vi "I(V) at various fields_MFLI_PK_v4.0_measure X.vi"() -> ()   [LabVIEW 2016]
uses:
  <instrlib>/Zurich Instruments LabOne/Public/Data/ziTypeDemodSampleSingle.ctl
  <instrlib>/Zurich Instruments LabOne/Public/Configure/ziSetValueDouble.vi
  <instrlib>/Zurich Instruments LabOne/Public/Configure/ziGetValueDemodSampleEx.vi
  <instrlib>/Zurich Instruments LabOne/Zurich Instruments LabOne.lvlib
panel:
  out "Time (s)":dbl format="%#_13g"
  in  "Field ramp rate (T/min)":string="0.05"
  in  "Magnetic field stabilization time (s)":dbl=200.0 format="%#_13g"
  in  "Step 2":dbl[](array[numeric])=[0.25] min=-3000.0 max=3000.0 format="%.1e"
  in  "To 2":dbl[](array[numeric])=[6.0] min=-3000.0 max=3000.0 format="%.1e"
  in  "From 2":dbl[](array[numeric])=[8.5] min=-3000.0 max=3000.0 format="%.1e"
  out "Magnetic Field (T)":dbl format="%#_13g"
  in  "Magnet IP Address":string="169.254.46.132"
  out "Demod Sample Out 2":T1={"Timestamps (ticks)"=34359738372, "X (Vrms)"=8.366245757779461e-285, "Y (Vrms)"=1.0096057436928657e-284, "Osc Phase (deg)"=1.69759663376e-313, "Freq (Hz)"=2.607691286315397e-191, "DIO"=4, "AuxIn0 (V)"=0.0, "AuxIn1 (V)"=1.6954746369817e-311, "Trigger"=16}
  out "Demod Sample Out":T1={"Timestamps (ticks)"=34359738372, "X (Vrms)"=8.366245757779461e-285, "Y (Vrms)"=1.0096057436928657e-284, "Osc Phase (deg)"=1.69759663376e-313, "Freq (Hz)"=2.607691286315397e-191, "DIO"=4, "AuxIn0 (V)"=0.0, "AuxIn1 (V)"=1.6954746369817e-311, "Trigger"=16}
  in  "MFLI Current source/Voltage reader":string="DEV4382"
  out "Imeas (A)":dbl=2.528615115e-315
  out "Vmeas (V)":dbl=nan
  in  "Folder":path=path "D:/Pranava/Data/NbO/27-05-2020"
  in  "MFLI stabilization time (s) [> TC]":u32=1
  out "I vs V":cluster{dbl, "Field Reading":dbl}[](graph)=[{nan, "Field Reading"=3.54694038e-315}, {nan, "Field Reading"=2.528615115e-315}]
  out "data":dbl[](array[numeric])=[nan, 2.528615115e-315, 0.0001]
  in  "Step":dbl[](array[numeric])=[0.001, 0.001, 0.001] min=-3000.0 max=3000.0 format="%.1e"
  in  "To":dbl[](array[numeric])=[0.5, -0.5, 0.0] min=-3000.0 max=3000.0 format="%.1e"
  in  "From":dbl[](array[numeric])=[0.0, 0.5, -0.5] min=-3000.0 max=3000.0 format="%.1e"
  in  "file name":string="001_IV_(Nb)STO_7mK_MFLI_MF-MD"
  out "File path":path=path "D:/Pranava/Data/001_IV_(Nb)STO_7mK_MFLI_MF-MD.dat"
  # ".dat"
  # "[Must be less than 0.05]"
  # "Set MFLI Voltage output (V)"
  # "Configure Magnetic field sweep (T)"
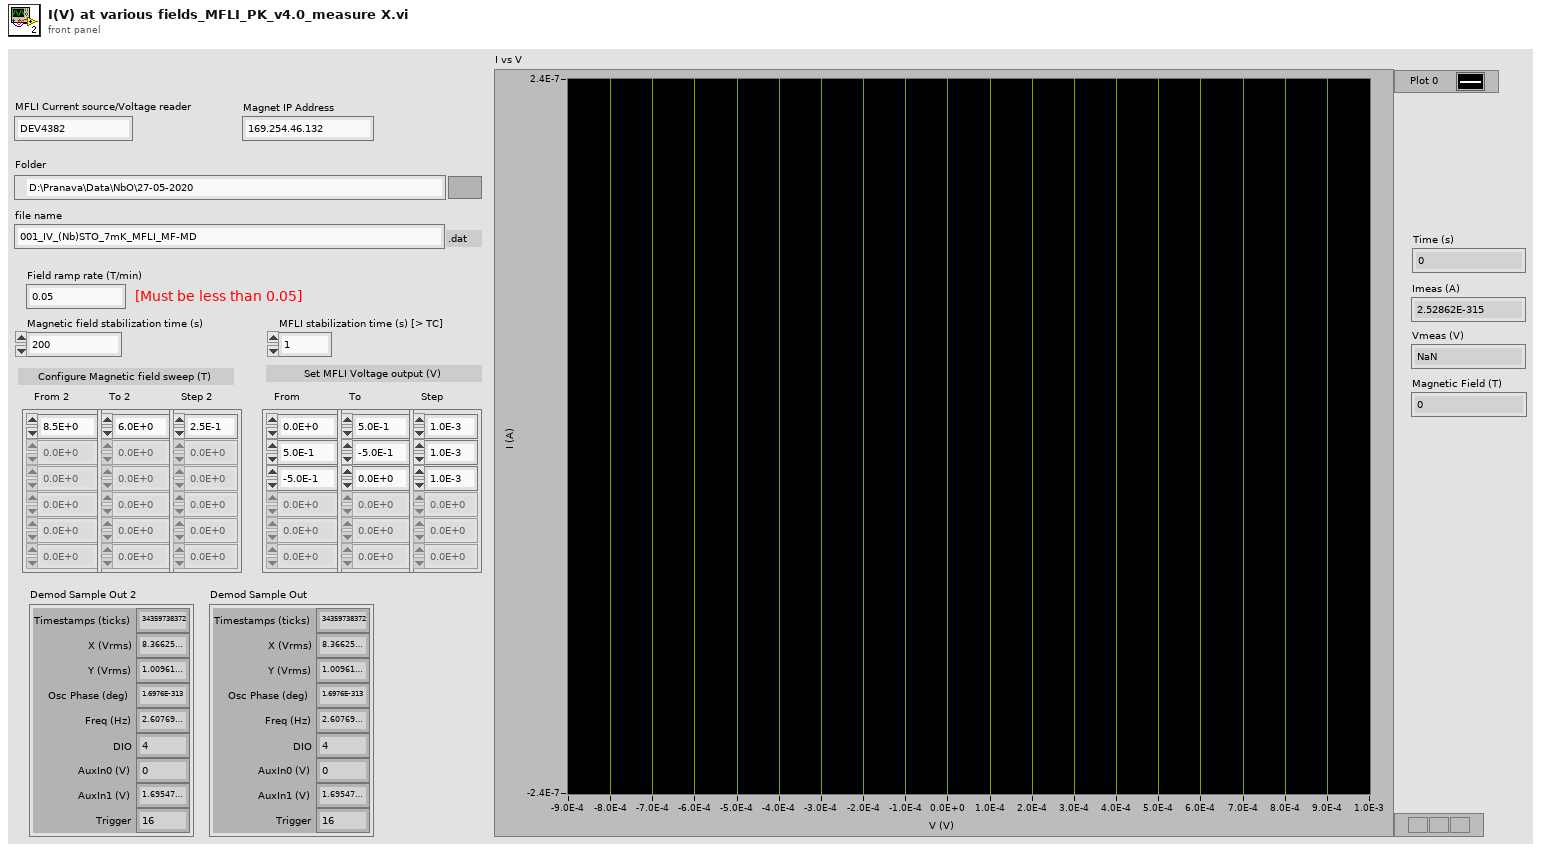
[diagram p1: front panel]
types:
  T1 = typedef "Zurich Instruments LabOne.lvlib/ziTypeDemodSampleSingle.ctl" = cluster{"Timestamps (ticks)":u64, "X (Vrms)":dbl, "Y (Vrms)":dbl, "Osc Phase (deg)":dbl, "Freq (Hz)":dbl, "DIO":u32, "AuxIn0 (V)":dbl, "AuxIn1 (V)":dbl, "Trigger":u32}
  T2 = enum16{"open", "replace", "create", "open or create", "replace or create", "replace or create with confirmation"}
  T3 = typedef "Zurich Instruments LabOne.lvlib/ziTypeHandle.ctl" = cluster{"handleValid":bool, "Conn":u64, "Path Prefix":string, "Handle":u64, "Connected":bool, "Clockbase(s)":dbl}
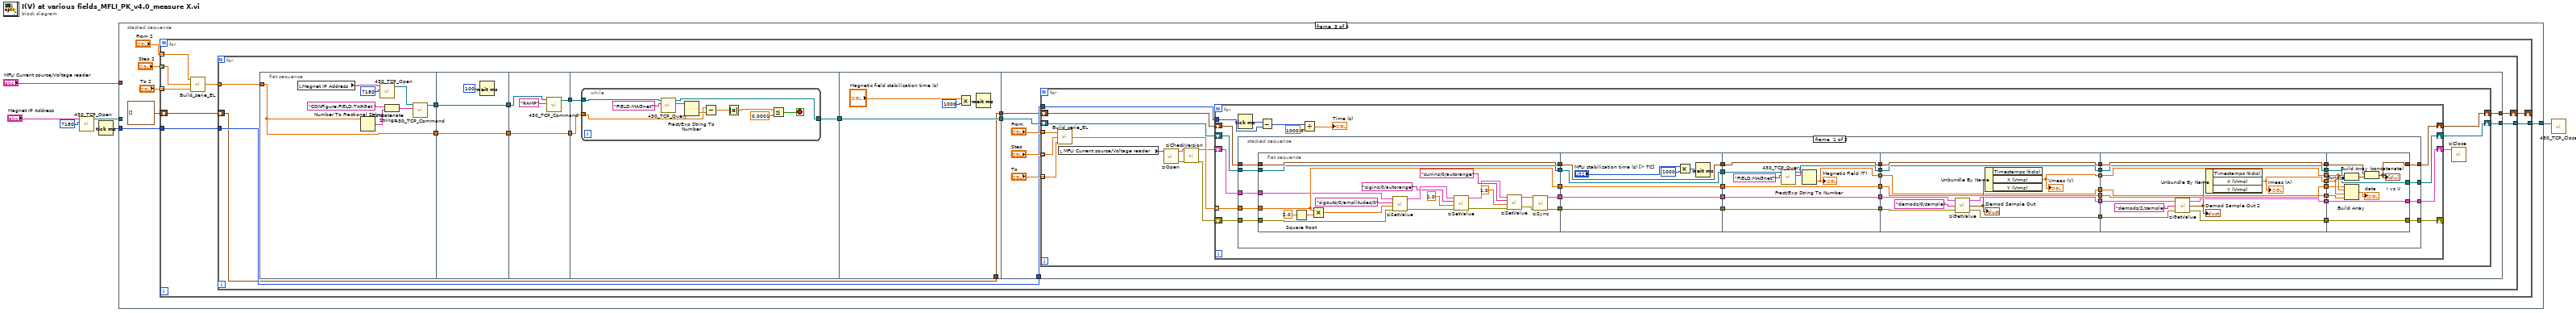
[diagram p0: block diagram]
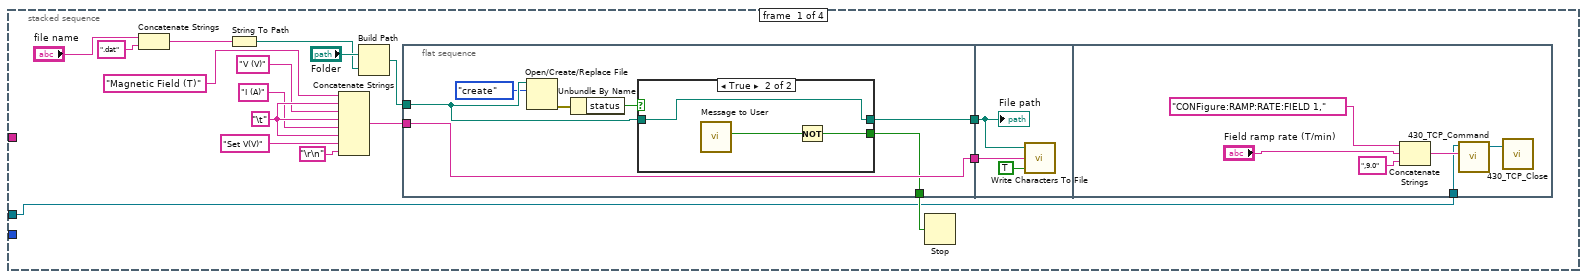
[diagram p2: hidden frame]
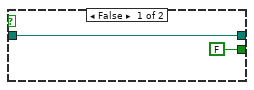
[diagram p3: hidden frame]
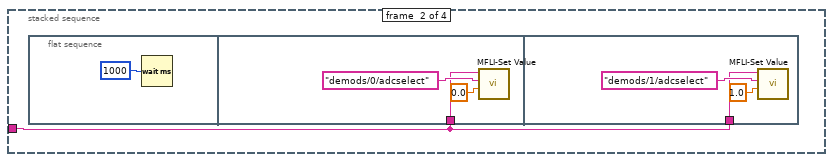
[diagram p4: hidden frame]
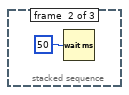
[diagram p5: hidden frame]
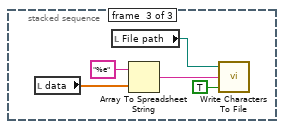
[diagram p6: hidden frame]
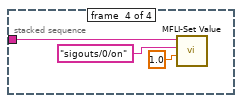
[diagram p7: hidden frame]
diagram:
  n1 = call "430_TCP_Open.vi"("IP Address"="Magnet IP Address", "TCP Port"=7180) -> ("connection ID"=w2:refnum<k5>)  [unwired: 4 in, 2 out]
  n2 = Tick Count (ms)() -> (millisecond timer value=w1:u32)
  n3 = stacked-sequence {
    tunnel: "MFLI Current source/Voltage reader" -> [_ w45 _ w269]
    tunnel: [_ _ w55 _] -> w5
    tunnel: w2 -> [w7 _ _ _]
    tunnel: w1 -> [_ _ w54 _]
    frame #0 {
      w20 = "\t"
      n4 = Concatenate Strings("file name", ".dat" ("string")) -> (w18:string)
      n5 = String To Path(string=w18) -> (path=w9:path)
      n6 = Concatenate Strings("Magnetic Field (T)", w20, "V (V)" ("string"), w20, "I (A)" ("string"), w20, "Set V(V)" ("string"), "\r\n") -> (w19:string)
      n7 = Build Path(base path="Folder", name or relative path=w9) -> (appended path=w8:path)
      n8 = flat-sequence {
        tunnel: w8 -> [w27]
        tunnel: w19 -> [w30]
        tunnel: [w30] -> w23
        tunnel: [w29] -> w16
        tunnel: [w28] -> w22
        tunnel: w23 -> [w37]
        tunnel: w22 -> [w36]
        tunnel: w7 -> [w39]
        frame #0 {
          n9 = Open/Create/Replace File(file path (use dialog)=w27, operation (0:open)=T2."create") -> (error out=w26:errorcluster)  [unwired: 4 in, 2 out]
          n10 = Unbundle By Name(w26) -> ("status"=w24:bool)
          n11 = case shown="True" w24 {
            tunnel: [FALSE ("Yes") w34] -> w29
            tunnel: [w31 w33] -> w28
            tunnel: w27 -> [w31 w33]
            frame False {
            }
            frame True {
              n12 = call "Message to User"() -> ("Yes"=w35:bool)  [unwired: 10 in, 1 out]
              n13 = Not(x=w35) -> (.not. x?=w34:bool)
            }
          }
        }
        frame #1 {
          n14 = call <vilib>:"Write Characters To File.vi"("append to file? (new file:F)"=TRUE, "character string"=w37, "file path (dialog if empty)"=w36) -> ()  [unwired: 2 in, 1 out]
          "File path" <- w36
        }
        frame #2 {
          n15 = Concatenate Strings("CONFigure:RAMP:RATE:FIELD 1," ("String"), "Field ramp rate (T/min)", ",9.0") -> (w40:string)
          n16 = call "430_TCP_Command.vi"("Command"=w40, "connection ID"=w39) -> ("connection ID out"=w44:refnum<k5>)  [unwired: 2 in, 2 out]
          n17 = call "430_TCP_Close.vi"("connection ID"=w44) -> ()  [unwired: 1 in, 2 out]
        }
      }
      n18 = Stop(stop? (T)=w16) -> ()
    }
    frame #1 {
      n19 = flat-sequence {
        tunnel: w45 -> [w47]
        tunnel: w45 -> [w50]
        frame #0 {
          n20 = Wait (ms)(milliseconds to wait=u32 1000) -> ()  [unwired: 1 out]
        }
        frame #1 {
          n21 = call "MFLI-Set Value.vi"("Value"=0.0, "Path"="demods/0/adcselect", "MFLI Current source/Voltage reader"=w47) -> ()  [unwired: 9 in]
        }
        frame #2 {
          n22 = call "MFLI-Set Value.vi"("Value"=1.0, "Path"="demods/1/adcselect", "MFLI Current source/Voltage reader"=w50) -> ()  [unwired: 9 in]
        }
      }
    }
    frame #2 {
      n23 = for {
        tunnel: "From 2" -> [w66] mode=indexing
        tunnel: "To 2" -> [w64] mode=indexing
        tunnel: "Step 2" -> [w65] mode=indexing
        tunnel: [w62] -> w55
        tunnel: w54 -> [w61]
        shift-right: [w59] -> _
        shift-left: cluster{dbl, "Field Reading":dbl}[] [] -> [w60]
        n24 = call "Build_serie_EL.vi"("end value"=w64, "increment"=w65, "start value"=w66) -> ("output array"=w63:dbl[])
        n25 = for {
          tunnel: w63 -> [w80] mode=indexing
          tunnel: [w75] -> w62
          tunnel: w61 -> [w70]
          shift-right: [w67] -> w59
          shift-left: w60 -> [w68]
          n26 = flat-sequence {
            tunnel: w80 -> [w84]
            tunnel: [w85] -> w74
            tunnel: [w84] -> w72
            tunnel: w74 -> [w91]
            tunnel: [w91] -> w73
            tunnel: w72 -> [w90]
            tunnel: [w90] -> w71
            tunnel: w73 -> [w95]
            tunnel: [w93] -> w79
            tunnel: [w92] -> w78
            tunnel: w71 -> [w92]
            tunnel: w79 -> [w98]
            tunnel: w78 -> [w97]
            tunnel: [w96] -> w76
            tunnel: [w110] -> w77
            tunnel: w76 -> [w110]
            tunnel: [w109] -> w69
            tunnel: w68 -> [w109]
            tunnel: w77 -> [w118]
            tunnel: [w117] -> w75
            tunnel: w70 -> [w116]
            tunnel: w69 -> [w115]
            tunnel: [w114] -> w67
            frame #0 {
              n27 = local read "Magnet IP Address"() -> (w82:string)
              n28 = Number To Fractional String(number=w84) -> (F-format string=w86:string)  [unwired: 3 in]
              n29 = call "430_TCP_Open.vi"("IP Address"=w82, "TCP Port"=7180) -> ("connection ID"=w81:refnum<k5>)  [unwired: 4 in, 2 out]
              n30 = Concatenate Strings("CONFigure:FIELD:TARGet " ("String"), w86) -> (w88:string)
              n31 = call "430_TCP_Command.vi"("Command"=w88, "connection ID"=w81) -> ("connection ID out"=w85:refnum<k5>)  [unwired: 2 in, 2 out]
            }
            frame #1 {
              n32 = Wait (ms)(milliseconds to wait=100) -> ()  [unwired: 1 out]
            }
            frame #2 {
              n33 = call "430_TCP_Command.vi"("Command"="RAMP", "connection ID"=w95) -> ("connection ID out"=w93:refnum<k5>)  [unwired: 2 in, 2 out]
            }
            frame #3 {
              n34 = while {
                tunnel: w98 -> [w108]
                tunnel: w97 -> [w103]
                tunnel: [w99] -> w96
                stop <- w101 stop-if-true
                n35 = call "430_TCP_Query.vi"("Command"="FIELD:MAGnet?" ("String"), "connection ID"=w108) -> ("Response"=w107:string, "connection ID out"=w99:refnum<k5>)  [unwired: 5 in, 3 out]
                n36 = Fract/Exp String To Number(string=w107) -> (number=w104:dbl)  [unwired: 3 in, 1 out]
                n37 = Subtract(x=w103, y=w104) -> (x-y=w106:dbl)
                n38 = Absolute Value(x=w106) -> (abs(x)=w105:dbl)
                n39 = Less Or Equal?(x=w105, y=0.0001) -> (x <= y?=w101:bool)
              }
            }
            frame #4 {
              n40 = Multiply(x="Magnetic field stabilization time (s)", y=1000) -> (x*y=w112:dbl)
              n41 = Wait (ms)(milliseconds to wait=w112) -> ()  [unwired: 1 out]
            }
            frame #5 {
              n42 = for {
                tunnel: "From" -> [w133] mode=indexing
                tunnel: "To" -> [w132] mode=indexing
                tunnel: "Step" -> [w131] mode=indexing
                shift-right: [w135] -> w114
                shift-left: w115 -> [w136]
                shift-right: [w123] -> w117
                shift-left: w118 -> [w124]
                tunnel: w116 -> [w122]
                n43 = call "Build_serie_EL.vi"("end value"=w132, "increment"=w131, "start value"=w133) -> ("output array"=w134:dbl[])
                n44 = local read "MFLI Current source/Voltage reader"() -> (w130:string)
                n45 = call <instrlib>:"ziOpen.vi"("Address"=w130) -> ("Error Out"=w129:errorcluster, "HandleOut"=w128:T3)  [unwired: 3 in, 1 out]
                n46 = call <instrlib>:"ziCheckVersion.vi"("Handle In"=w128, "Error In"=w129) -> ("Handle Out"=w127:T3, "Error Out"=w125:errorcluster)  [unwired: 11 in, 1 out]
                n47 = for {
                  tunnel: w134 -> [w150] mode=indexing
                  shift-right: [w148] -> w135
                  shift-left: w136 -> [w149]
                  shift-right: [w145] -> w126
                  shift-left: w127 -> [w147]
                  shift-right: [w144] -> _
                  shift-left: w125 -> [w146]
                  shift-right: [w143] -> w123
                  shift-left: w124 -> [w142]
                  tunnel: w122 -> [w138]
                  n48 = Tick Count (ms)() -> (millisecond timer value=w139:u32)
                  n49 = stacked-sequence {
                    tunnel: w150 -> [w188 _ _]
                    tunnel: w149 -> [w189 _ _]
                    tunnel: [w190 _ _] -> w148
                    tunnel: w147 -> [w183 _ _]
                    tunnel: w146 -> [w182 _ _]
                    tunnel: [w172 _ _] -> w145
                    tunnel: [w171 _ _] -> w144
                    tunnel: [w154 _ _] -> w143
                    tunnel: w142 -> [w153 _ _]
                    frame #0 {
                      n50 = flat-sequence {
                        tunnel: [w211] -> w187
                        tunnel: [w210] -> w186
                        tunnel: w188 -> [w210]
                        tunnel: w189 -> [w211]
                        tunnel: [w192] -> w185
                        tunnel: [w193] -> w184
                        tunnel: w183 -> [w195]
                        tunnel: w182 -> [w194]
                        tunnel: w153 -> [w191]
                        tunnel: [w191] -> w152
                        tunnel: w187 -> [w219]
                        tunnel: [w219] -> w164
                        tunnel: w186 -> [w218]
                        tunnel: [w218] -> w162
                        tunnel: [w217] -> w166
                        tunnel: [w216] -> w168
                        tunnel: w185 -> [w216]
                        tunnel: w184 -> [w217]
                        tunnel: w152 -> [w215]
                        tunnel: [w215] -> w151
                        tunnel: w168 -> [w228]
                        tunnel: [w228] -> w167
                        tunnel: w166 -> [w227]
                        tunnel: [w227] -> w165
                        tunnel: w164 -> [w226]
                        tunnel: [w226] -> w163
                        tunnel: w162 -> [w225]
                        tunnel: [w225] -> w161
                        tunnel: [w222] -> w158
                        tunnel: [w221] -> w157
                        tunnel: w151 -> [w220]
                        tunnel: [w231] -> w181
                        tunnel: [w239] -> w179
                        tunnel: [w238] -> w177
                        tunnel: w167 -> [w235]
                        tunnel: w165 -> [w234]
                        tunnel: w163 -> [w239]
                        tunnel: w161 -> [w238]
                        tunnel: [w233] -> w175
                        tunnel: [w232] -> w174
                        tunnel: [w230] -> w159
                        tunnel: w158 -> [w230]
                        tunnel: w157 -> [w229]
                        tunnel: [w229] -> w155
                        tunnel: w181 -> [w243]
                        tunnel: [w243] -> w180
                        tunnel: w179 -> [w251]
                        tunnel: [w251] -> w178
                        tunnel: w177 -> [w250]
                        tunnel: [w250] -> w176
                        tunnel: w175 -> [w247]
                        tunnel: w174 -> [w246]
                        tunnel: [w245] -> w173
                        tunnel: [w244] -> w170
                        tunnel: [w242] -> w169
                        tunnel: [w241] -> w160
                        tunnel: w159 -> [w241]
                        tunnel: [w240] -> w156
                        tunnel: w155 -> [w240]
                        tunnel: w180 -> [w261]
                        tunnel: [w260] -> w190
                        tunnel: w178 -> [w259]
                        tunnel: w176 -> [w258]
                        tunnel: [w257] -> w172
                        tunnel: w173 -> [w257]
                        tunnel: [w256] -> w171
                        tunnel: w170 -> [w256]
                        tunnel: w169 -> [w255]
                        tunnel: w160 -> [w253]
                        tunnel: w156 -> [w252]
                        tunnel: [w252] -> w154
                        frame #0 {
                          n51 = Square Root(x=2.0) -> (sqrt(x)=w209:dbl)
                          n52 = Multiply(x=w210, y=w209) -> (x*y=w206:dbl)
                          n53 = call-poly <instrlib>:"ziSetValue.vi"("Error In"=w194, "Value"=w206, "Path"="sigouts/0/amplitudes/0", "Handle In"=w195) -> ("Error Out"=w202:errorcluster, "Handle Out"=w205:T3)  [unwired: 1 in]
                          n54 = call-poly <instrlib>:"ziSetValue.vi"("Error In"=w202, "Value"=1.0, "Path"="sigins/0/autorange", "Handle In"=w205) -> ("Error Out"=w198:errorcluster, "Handle Out"=w199:T3)  [unwired: 1 in]
                          n55 = call-poly <instrlib>:"ziSetValue.vi"("Error In"=w198, "Value"=1.0, "Path"="currins/0/autorange", "Handle In"=w199) -> ("Error Out"=w196:errorcluster, "Handle Out"=w197:T3)  [unwired: 1 in]
                          n56 = call <instrlib>:"ziSync.vi"("Handle In"=w197, "Error In"=w196) -> ("Handle Out"=w193:T3, "Error Out"=w192:errorcluster)  [unwired: 12 in]
                        }
                        frame #1 {
                          n57 = Multiply(x="MFLI stabilization time (s) [> TC]", y=1000) -> (x*y=w213:u32)
                          n58 = Wait (ms)(milliseconds to wait=w213) -> ()  [unwired: 1 out]
                        }
                        frame #2 {
                          n59 = call "430_TCP_Query.vi"("Command"="FIELD:MAGnet?" ("String"), "connection ID"=w220) -> ("Response"=w224:string, "connection ID out"=w221:refnum<k5>)  [unwired: 5 in, 3 out]
                          n60 = Fract/Exp String To Number(string=w224) -> (number=w222:dbl)  [unwired: 3 in, 1 out]
                          "Magnetic Field (T)" <- w222
                        }
                        frame #3 {
                          n61 = call-poly <instrlib>:"ziGetValue.vi"("error in"=w235, "Path"="demods/0/sample", "Handle In"=w234) -> ("error out"=w232:errorcluster, "Demod Sample Out"=w236:T1, "Handle Out"=w233:T3)
                          "Demod Sample Out" <- w236
                          n62 = Unbundle By Name(w236) -> ("X (Vrms)"=w231:dbl)  [unwired: 2 out]
                          "Vmeas (V)" <- w231
                        }
                        frame #4 {
                          n63 = call-poly <instrlib>:"ziGetValue.vi"("error in"=w246, "Path"="demods/2/sample", "Handle In"=w247) -> ("error out"=w244:errorcluster, "Demod Sample Out"=w248:T1, "Handle Out"=w245:T3)
                          "Demod Sample Out 2" <- w248
                          n64 = Unbundle By Name(w248) -> ("X (Vrms)"=w242:dbl)  [unwired: 2 out]
                          "Imeas (A)" <- w242
                        }
                        frame #5 {
                          n65 = Bundle("X (Vrms)"=w261, "X (Vrms)"=w255) -> (w254:cluster{"X (Vrms)":dbl, "X (Vrms)":dbl})  [unwired: 1 in]
                          n66 = Build Array(w253, w261, w255, w258) -> (→"data":dbl[])
                          n67 = Build Array (concatenate)(w259, w254) -> (w260:cluster{"X (Vrms)":dbl, "X (Vrms)":dbl}[])
                          "I vs V" <- w260
                        }
                      }
                    }
                    frame #1 {
                      n68 = Wait (ms)(milliseconds to wait=u32 50) -> ()  [unwired: 1 out]
                    }
                    frame #2 {
                      n69 = local read "data"() -> (w264:dbl[])
                      n70 = local read "File path"() -> (w266:path)
                      n71 = Array To Spreadsheet String(array=w264, 3:"%e" ("format string")) -> (spreadsheet string=w267:string)  [unwired: 1 in]
                      n72 = call <vilib>:"Write Characters To File.vi"("append to file? (new file:F)"=TRUE, "character string"=w267, "file path (dialog if empty)"=w266) -> ()  [unwired: 2 in, 1 out]
                    }
                  }
                  n73 = Subtract(x=w139, y=w138) -> (x-y=w141:u32)
                  n74 = Divide(x=w141, y=1000.0) -> (x/y=→"Time (s)":dbl)
                }
                n75 = call <instrlib>:"ziClose.vi"("Handle In"=w126) -> ()  [unwired: 1 in, 4 out]
              }
            }
          }
        }
      }
    }
    frame #3 {
      n76 = call "MFLI-Set Value.vi"("Value"=1.0, "Path"="sigouts/0/on", "MFLI Current source/Voltage reader"=w269) -> ()  [unwired: 9 in]
    }
  }
  n77 = call "430_TCP_Close.vi"("connection ID"=w5) -> ()  [unwired: 1 in, 2 out]
